vi "timer-state-machine.vi"() -> ()   [LabVIEW 2025]
panel:
  out "Seconds Elapsed":dbl
  out "Iteration":i32
  in  "Toggle":bool
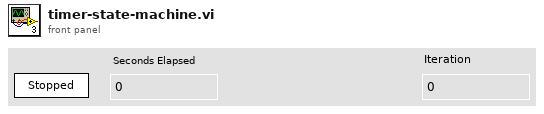
[diagram p1: front panel]
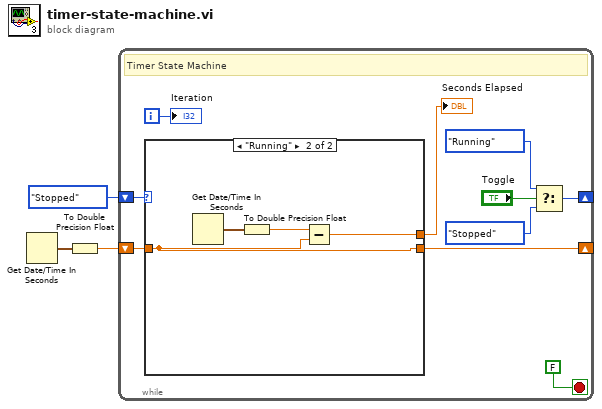
[diagram p0: block diagram]
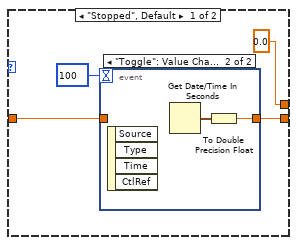
[diagram p2: hidden frame]
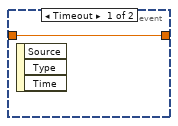
[diagram p3: hidden frame]
diagram:
  n1 = Get Date/Time In Seconds() -> (seconds since 1Jan1904=w1:timestamp)
  n2 = To Double Precision Float(number=w1) -> (double precision float=w2:dbl)
  n3 = while {
    shift-right: [w8] -> _
    shift-left: enum16{"Stopped", "Running"}."Stopped" -> [w13]
    shift-right: [w5] -> _
    shift-left: w2 -> [w12]
    i -> [w11]
    stop <- FALSE stop-if-true
    # "Timer State Machine"
    n4 = case shown="\"Running\"" w13 {
      tunnel: w12 -> [w14 w23]
      tunnel: [w16 w23] -> w5
      tunnel: [0.0 w21] -> w4
      frame "Stopped", Default {
        n5 = event shown="[1] \"Toggle\": Value Change" {
          selector: _ -> [_ _]
          dyn-events: _ -> [_ _]
          timeout: 100 -> [_ _]
          tunnel: [w18 w19] -> w16
          tunnel: w14 -> [w18 _]
          event Timeout {
            n6 = event-data() -> ()  [unwired: 1 in, 3 out]
          }
          event "Toggle": Value Change {
            n7 = event-data() -> ()  [unwired: 1 in, 4 out]
            n8 = Get Date/Time In Seconds() -> (seconds since 1Jan1904=w20:timestamp)
            n9 = To Double Precision Float(number=w20) -> (double precision float=w19:dbl)
          }
        }
      }
      frame "Running" {
        n10 = Get Date/Time In Seconds() -> (seconds since 1Jan1904=w24:timestamp)
        n11 = To Double Precision Float(number=w24) -> (double precision float=w22:dbl)
        n12 = Subtract(x=w22, y=w23) -> (x-y=w21:dbl)
      }
    }
    "Seconds Elapsed" <- w4
    n13 = Select(t=enum16{"Stopped", "Running"}."Running", s="Toggle", f=enum16{"Stopped", "Running"}."Stopped") -> (s? t:f=w8:enum16{"Stopped", "Running"})
    "Iteration" <- w11
  }
